vi "003_petlaZdarzenStat_MG.vi"() -> ()   [LabVIEW 2021]
uses:
  <vilib>/Analysis/baseanly.llb/Mean (DBL).vi
  <vilib>/Analysis/NI_AALBase.lvlib
panel:
  in  "Reset":bool
  out "Najkrótszy czas":dbl=0.338
  out "Najdłuższy czas":dbl=14.05
  out "Średni czas":dbl=1.2933124999999999 format="%0.2f"
  out "Waveform Graph":dbl[](graph)=[0.648, 0.579, 0.552, 0.474, 0.344, 0.348, 0.354, 0.411, 0.393, 0.395, 0.467, 0.389, 0.532, 0.338, 0.419, 14.05]
  out "Procent":dbl=88.88888888888889
  out "Ilość prób":i32=18
  out "Kombinacja":u32=3
  out "Oczekiwanie":u32=4675
  out "Czas start":u32=16961757
  out "Poprawana reakcja?":string="Tak"
  out "Czas reakcji [s]":dbl=14.05
  out "Prawa":bool=TRUE
  out "Lewa":bool
  in  "Start":bool
  in  "3":bool
  in  "2":bool
  in  "1":bool
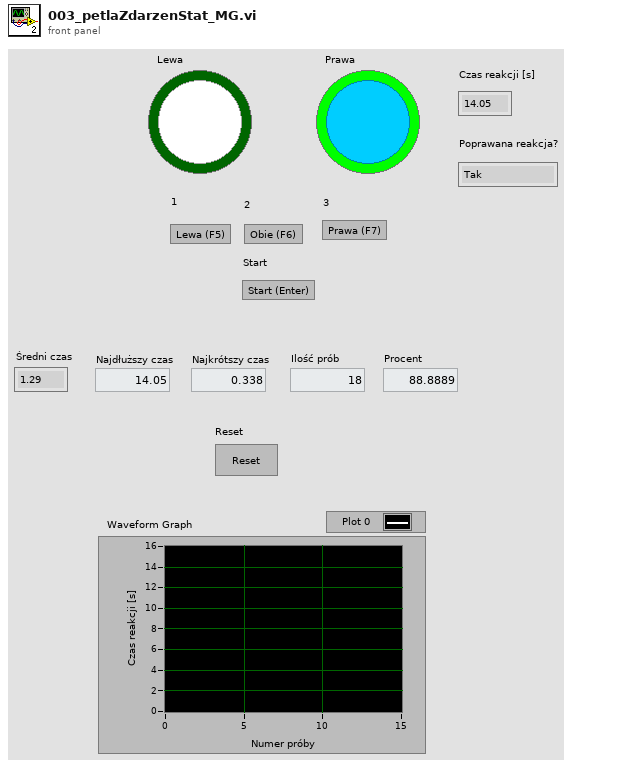
[diagram p1: front panel]
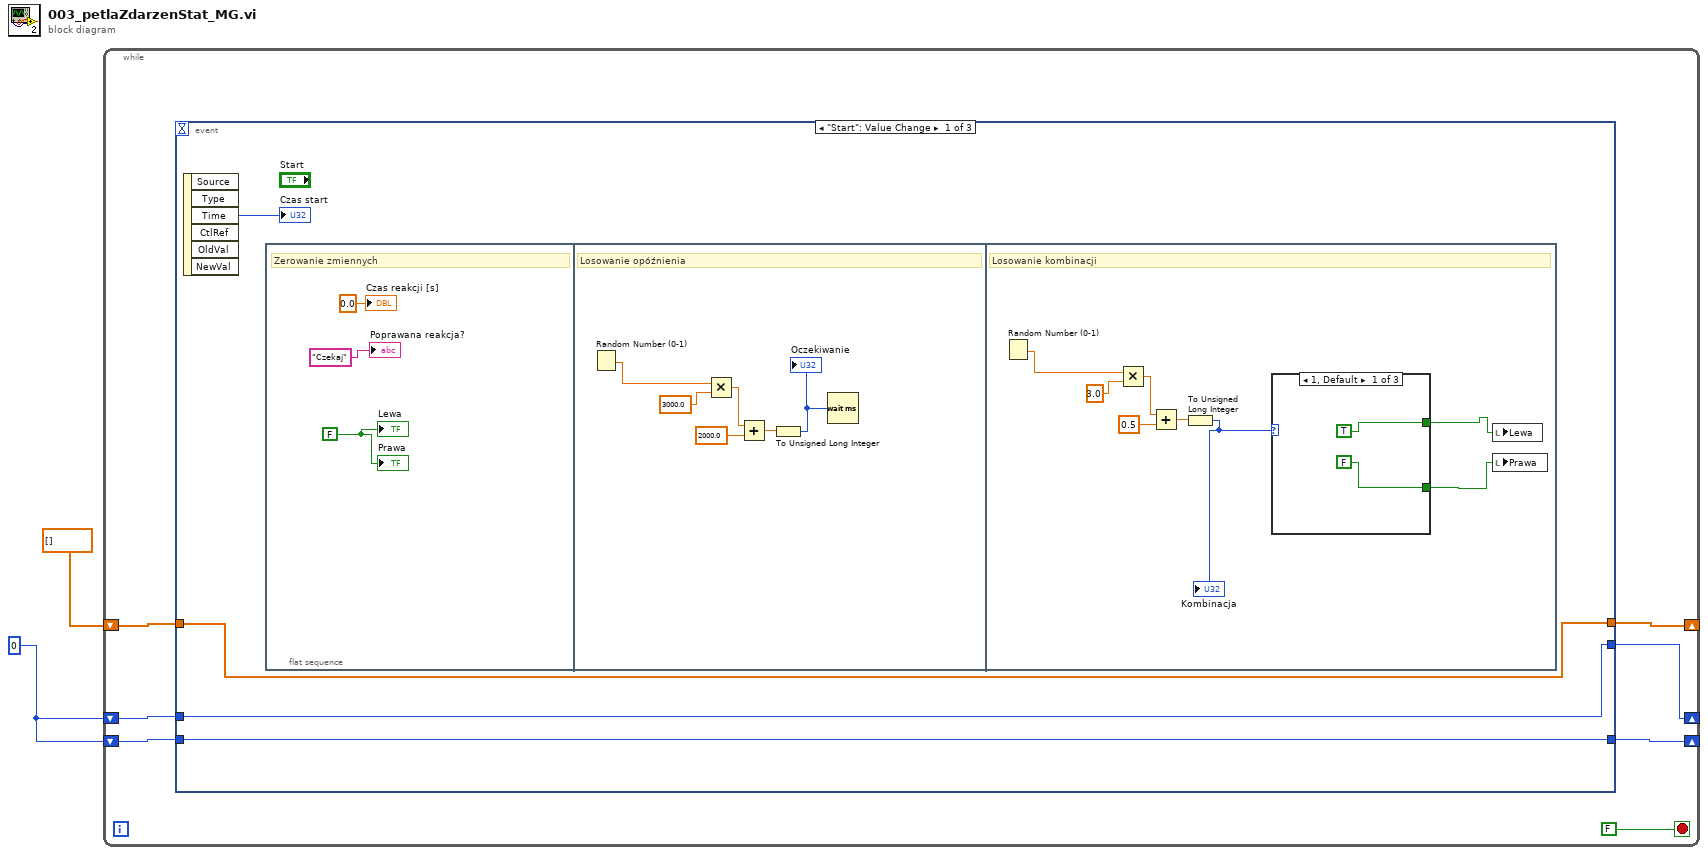
[diagram p0: block diagram]
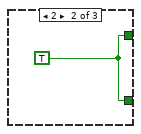
[diagram p2: hidden frame]
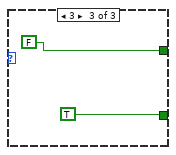
[diagram p3: hidden frame]
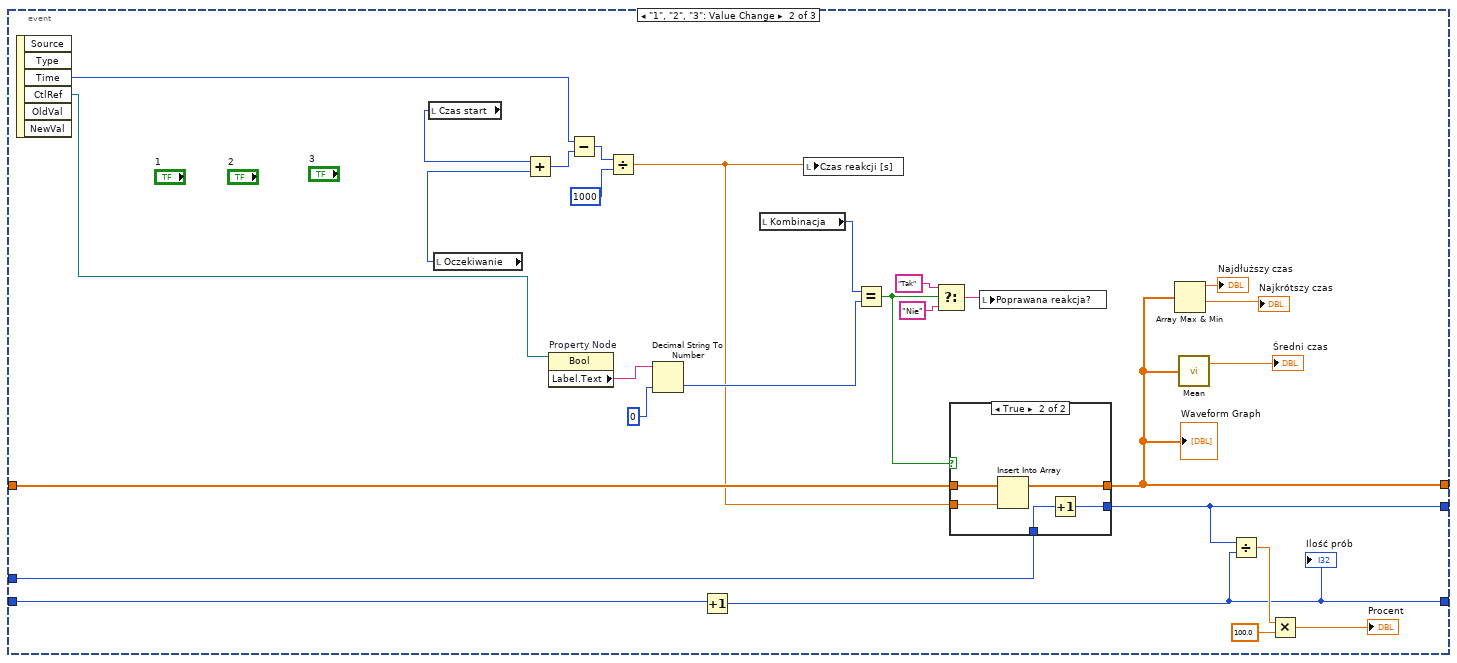
[diagram p4: hidden frame]
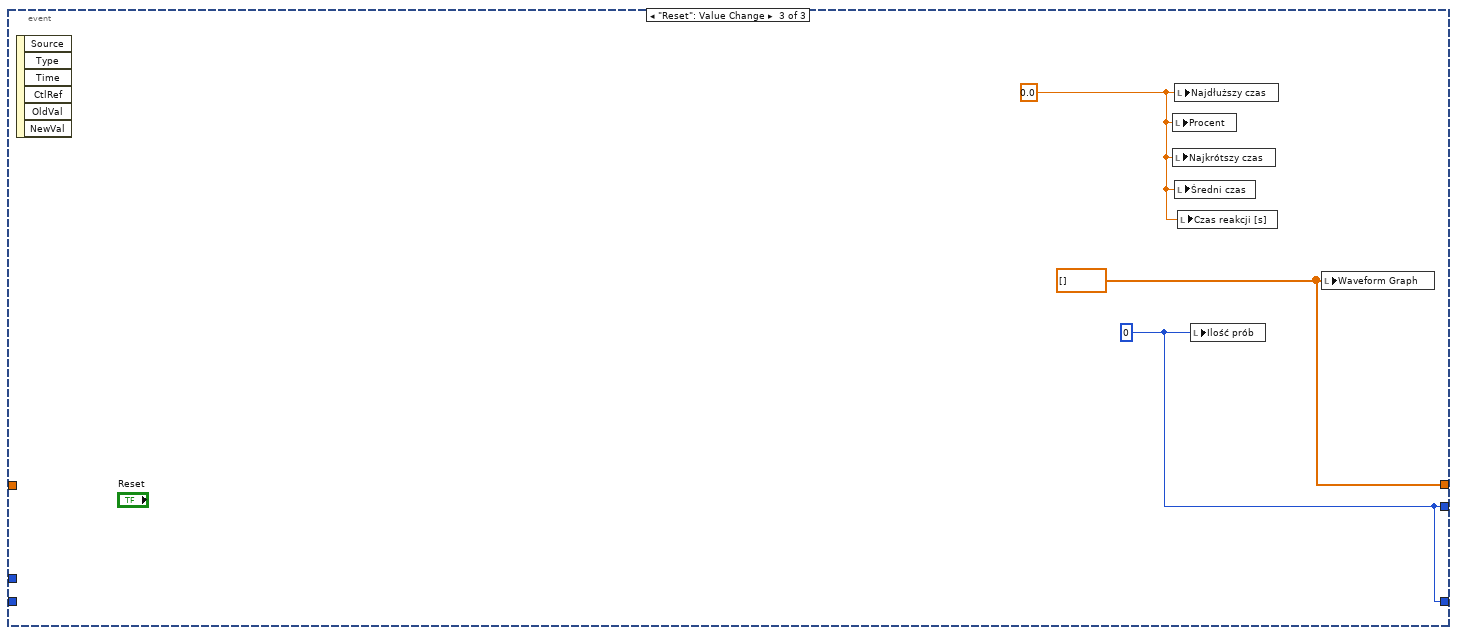
[diagram p6: hidden frame]
diagram:
  w1 = 0
  n1 = while {
    shift-right: [w3] -> _
    shift-left: dbl[] [] ("array") -> [w8]
    shift-right: [w6] -> _
    shift-left: w1 -> [w7]
    shift-right: [w4] -> _
    shift-left: w1 -> [w5]
    stop <- FALSE stop-if-true
    n2 = event shown="[0] \"Start\": Value Change" {
      selector: _ -> [_ _ _]
      dyn-events: _ -> [_ _ _]
      timeout: _ -> [_ _ _]
      tunnel: w8 -> [w12 w48 _]
      tunnel: w7 -> [w11 w46 _]
      tunnel: [w11 w45 w71] -> w6
      tunnel: w5 -> [w10 w37 _]
      tunnel: [w10 w36 w71] -> w4
      tunnel: [w12 w40 w72] -> w3
      event "Start": Value Change {
        n3 = event-data() -> ("Time"=→"Czas start":u32)  [unwired: 1 in, 5 out]
        n4 = flat-sequence {
          frame #0 {
            w14 = FALSE ("Lewa")
            # "Zerowanie zmiennych"
            "Poprawana reakcja?" <- "Czekaj" ("Poprawana reakcja?")
            "Czas reakcji [s]" <- 0.0 ("Czas reakcji [s]")
            "Lewa" <- w14
            "Prawa" <- w14
          }
          frame #1 {
            # "Losowanie opóźnienia"
            n5 = Random Number (0-1)() -> (number: 0 to 1=w22:dbl)
            n6 = Multiply(x=w22, y=3000.0) -> (x*y=w20:dbl)
            n7 = Add(x=w20, y=2000.0) -> (x+y=w18:dbl)
            n8 = To Unsigned Long Integer(number=w18) -> (unsigned 32bit integer=w17:u32)
            "Oczekiwanie" <- w17
            n9 = Wait (ms)(milliseconds to wait=w17) -> ()  [unwired: 1 out]
          }
          frame #2 {
            # "Losowanie kombinacji"
            n10 = Random Number (0-1)() -> (number: 0 to 1=w30:dbl)
            n11 = Multiply(x=w30, y=3.0) -> (x*y=w28:dbl)
            n12 = Add(x=w28, y=0.5) -> (x+y=w26:dbl)
            n13 = To Unsigned Long Integer(number=w26) -> (unsigned 32bit integer=w25:u32)
            "Kombinacja" <- w25
            n14 = case shown="1, Default" w25 {
              tunnel: [TRUE w33 FALSE] -> w24
              tunnel: [FALSE w33 TRUE] -> w23
              frame 1, Default {
              }
              frame 2 {
                w33 = TRUE
              }
              frame 3 {
              }
            }
            n15 = local write "Lewa"(w24) -> ()
            n16 = local write "Prawa"(w23) -> ()
          }
        }
      }
      event "1", "2", "3": Value Change {
        n17 = event-data() -> ("Time"=w60:u32, "CtlRef"=w57:refnum<vi>)  [unwired: 1 in, 4 out]
        n18 = local read "Czas start"() -> (w62:u32)
        n19 = local read "Oczekiwanie"() -> (w61:u32)
        n20 = Add(x=w62, y=w61) -> (x+y=w63:u32)
        n21 = property on="Property Node" class="Bool"(reference=w57) -> ("Label.Text"=w56:string)  [unwired: 1 in, 2 out]
        n22 = Subtract(x=w60, y=w63) -> (x-y=w59:u32)
        n23 = Divide(x=w59, y=u32 1000) -> (x/y=w47:dbl)
        n24 = Decimal String To Number(string=w56, default (0L)=u8 0 ("default (0 I32)")) -> (number=w54:u8)  [unwired: 1 in, 1 out]
        n25 = Increment(x=w37) -> (x+1=w36:i32)
        "Ilość prób" <- w36
        n26 = local read "Kombinacja"() -> (w53:u32)
        n27 = local write "Czas reakcji [s]"(w47) -> ()
        n28 = Equal?(x=w53, y=w54) -> (x = y?=w49:bool)
        n29 = Select(t="Tak", s=w49, f="Nie") -> (s? t:f=w50:string)
        n30 = case shown="True" w49 {
          tunnel: w48 -> [w65 w70]
          tunnel: w47 -> [_ w69]
          tunnel: w46 -> [w64 w68]
          tunnel: [w64 w67] -> w45
          tunnel: [w65 w66] -> w40
          frame False {
          }
          frame True {
            n31 = Insert Into Array(array=w70, new element=w69) -> (w66:dbl[])  [unwired: 1 in]
            n32 = Increment(x=w68) -> (x+1=w67:i32)
          }
        }
        "Waveform Graph" <- w40
        n33 = local write "Poprawana reakcja?"(w50) -> ()
        n34 = Array Max & Min(array=w40) -> (max value=→"Najdłuższy czas":dbl, min value=→"Najkrótszy czas":dbl)  [unwired: 2 out]
        n35 = call-poly <vilib>:"Mean.vi"("X"=w40) -> ("mean"=→"Średni czas":dbl)  [unwired: 1 out]
        n36 = Divide(x=w45, y=w36) -> (x/y=w44:dbl)
        n37 = Multiply(x=w44, y=100.0) -> (x*y=→"Procent":dbl)
      }
      event "Reset": Value Change {
        w71 = 0 ("Ilość prób")
        w73 = 0.0 ("Najdłuższy czas")
        w72 = dbl[] [] ("array")
        n38 = event-data() -> ()  [unwired: 1 in, 6 out]
        n39 = local write "Procent"(w73) -> ()
        n40 = local write "Najkrótszy czas"(w73) -> ()
        n41 = local write "Najdłuższy czas"(w73) -> ()
        n42 = local write "Średni czas"(w73) -> ()
        n43 = local write "Czas reakcji [s]"(w73) -> ()
        n44 = local write "Ilość prób"(w71) -> ()
        n45 = local write "Waveform Graph"(w72) -> ()
      }
    }
  }
